vi "Set Dual Exposure Times.vi"(10 "expTime2":sgl, 11 "expTime1":sgl) -> (3 "function return":u32)   [LabVIEW 2018, in "Copy of Andor SDK.lvlib"]
doc: "EXPNETTYPE unsigned int WINAPI SetDualExposureTimes(float expTime1, float expTime2);"
uses:
  Copy of Andor SDK.lvlib
  <userlib>/Andor SDK/ATMCD32D.dll
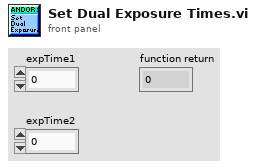
[diagram p1: front panel]
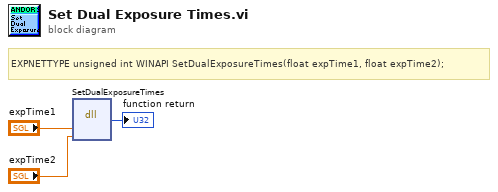
[diagram p0: block diagram]
diagram:
  # "EXPNETTYPE unsigned int WINAPI SetDualExposureTimes(float expTime1, float expTime2);"
  n1 = dll-call lib="C:/Program Files (x86)/National Instruments/LabVIEW 2018/user.lib/Andor SDK/ATMCD32D.*" fn="SetDualExposureTimes"("expTime1"="expTime1", "expTime2"="expTime2") -> (→"function return":u32)  [unwired: 5 in, 2 out]
